vi "counter_channel_producer_with_max_count.vi"(7 "Channel":i32, 8 "error in (no error)":errorcluster, 9 "aData Out":dbl[][](array[numeric]), 10 "Queue in":refnum<queue>, 11 "output cluster in":T1) -> (0 "error out":errorcluster, 3 "output cluster out":T1)   [LabVIEW 2025, in "LabJackEKG.lvlib"]
uses:
  LabJackEKG.lvlib
  Tests/StreamProducerLoopData.ctl
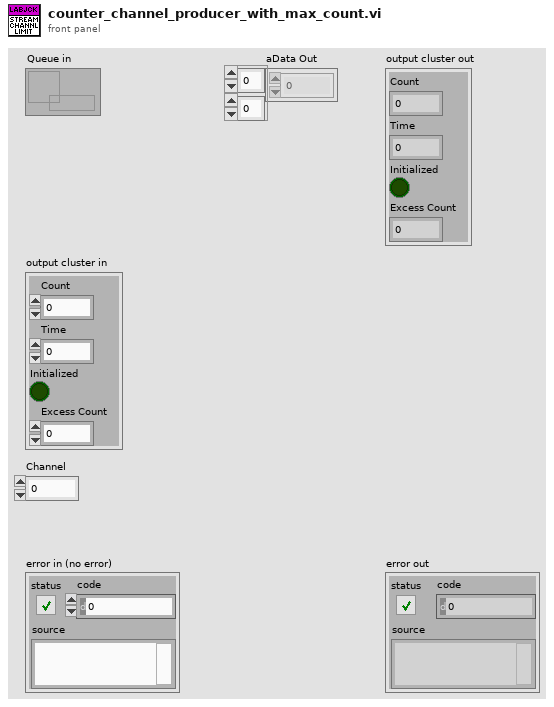
[diagram p1: front panel]
types:
  T1 = typedef "LabJackEKG.lvlib/StreamProducerLoopData.ctl" = cluster{"Count":i64, "Time":i64, "Initialized":bool, "Excess Count":i64}
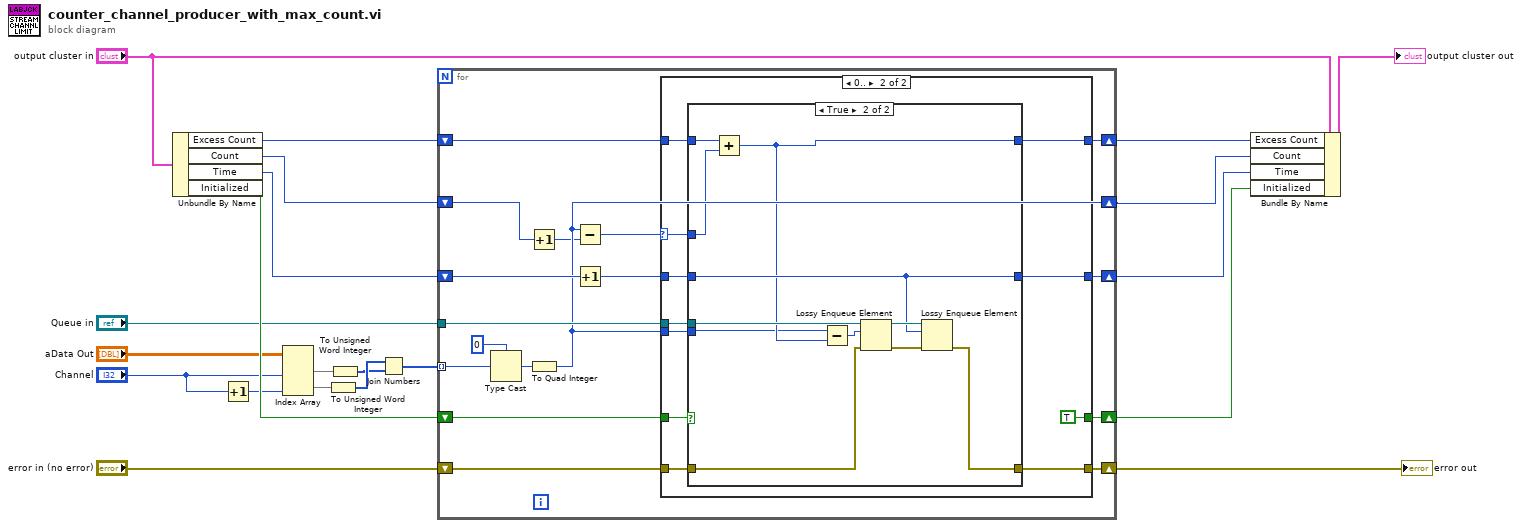
[diagram p0: block diagram]
diagram:
  n1 = Unbundle By Name("output cluster in") -> ("Excess Count"=w2:i64, "Count"=w21:i64, "Time"=w20:i64, "Initialized"=w19:bool)
  n2 = Increment(x="Channel") -> (x+1=w6:i32)
  n3 = Index Array(array="aData Out", index (col) #1="Channel", index (col) #2=w6) -> (element #1=w9:dbl[], element #2=w13:dbl[])  [unwired: 2 in]
  n4 = To Unsigned Word Integer(number=w13) -> (unsigned 16bit integer=w5:u16[])
  n5 = To Unsigned Word Integer(number=w9) -> (unsigned 16bit integer=w4:u16[])
  n6 = Join Numbers(hi=w5, lo=w4) -> ((hi.lo)=w3:u32[])
  n7 = for {
    tunnel: w3 -> [w33] mode=indexing
    tunnel: "Queue in" -> [w38]
    shift-right: [w37] -> w12
    shift-left: "error in (no error)" -> [w36]
    shift-right: [w35] -> w15
    shift-left: w20 -> [w34]
    shift-right: [w27] -> w14
    shift-left: w21 -> [w23]
    shift-right: [w31] -> w16
    shift-left: w19 -> [w30]
    shift-right: [w24] -> w1
    shift-left: w2 -> [w25]
    n8 = Type Cast(type=0, x=w33) -> (*(type *) &x=w29:i32)
    n9 = Increment(x=w23) -> (x+1=w22:i64)
    n10 = To Quad Integer(1:w29) -> (0:w27:i64)
    n11 = Subtract(x=w27, y=w22) -> (x-y=w26:i64)
    n12 = Increment(x=w34) -> (x+1=w32:i64)
    n13 = case shown="0.." w26 {
      selector: w26 -> [_ w43]
      tunnel: w38 -> [_ w53]
      tunnel: [w42 w50] -> w37
      tunnel: w36 -> [w42 w52]
      tunnel: w27 -> [_ w51]
      tunnel: [w41 w46] -> w35
      tunnel: w32 -> [w41 w49]
      tunnel: [w40 TRUE] -> w31
      tunnel: w30 -> [w40 w47]
      tunnel: w25 -> [w39 w45]
      tunnel: [w39 w44] -> w24
      frame Default {
      }
      frame 0.. {
        n14 = case shown="True" w47 {
          tunnel: w53 -> [_ w67]
          tunnel: w52 -> [w56 w65]
          tunnel: w51 -> [_ w58]
          tunnel: [w56 w64] -> w50
          tunnel: w49 -> [w55 w62]
          tunnel: [w55 w62] -> w46
          tunnel: w45 -> [w54 w61]
          tunnel: [w54 w59] -> w44
          tunnel: w43 -> [_ w60]
          frame False {
          }
          frame True {
            n15 = Add(x=w61, y=w60) -> (x+y=w59:i64)
            n16 = Subtract(x=w58, y=w59) -> (x-y=w57:i64)
            n17 = Lossy Enqueue Element(queue=w67, element=w57, error in (no error)=w65) -> (queue out=w63:refnum<queue>, error out=w66:errorcluster)  [unwired: 2 out]
            n18 = Lossy Enqueue Element(queue=w63, element=w62, error in (no error)=w66) -> (error out=w64:errorcluster)  [unwired: 3 out]
          }
        }
      }
    }
  }
  "error out" <- w12
  n19 = Bundle By Name(cluster="output cluster in", "Excess Count"=w1, "Count"=w14, "Time"=w15, "Initialized"=w16) -> (→"output cluster out":T1)
